vi "CheckStoped.vi"(0 "OSC in":refnum<visa-resource-name>, 1 "error in (no error)":errorcluster) -> (2 "OSC out":refnum<visa-resource-name>, 3 "Stopped?":bool, 4 "error out":errorcluster)   [LabVIEW 2016]
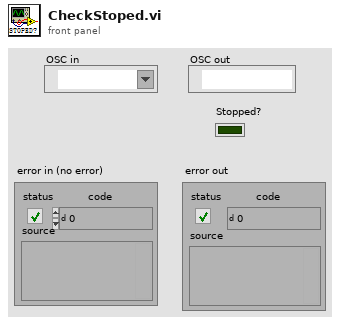
[diagram p1: front panel]
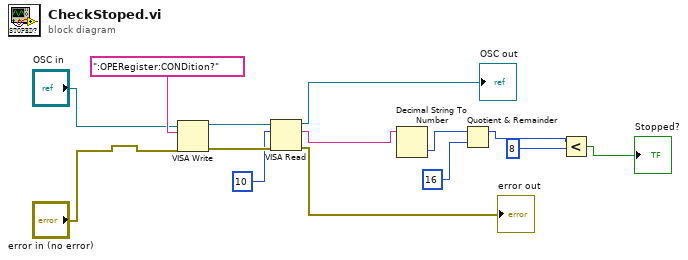
[diagram p0: block diagram]
diagram:
  n1 = VISA Write(VISA resource name="OSC in", write buffer=":OPERegister:CONDition?", error in (no error)="error in (no error)") -> (VISA resource name out=w13:refnum<visa-resource-name>, error out=w12:errorcluster)  [unwired: 1 out]
  n2 = VISA Read(VISA resource name=w13, byte count=10, error in (no error)=w12) -> (VISA resource name out=→"OSC out":refnum<visa-resource-name>, read buffer=w8:string, error out=→"error out":errorcluster)  [unwired: 1 out]
  n3 = Decimal String To Number(string=w8) -> (number=w7:i32)  [unwired: 2 in, 1 out]
  n4 = Quotient & Remainder(x=w7, y=16) -> (x-y*floor(x/y)=w5:i32)  [unwired: 1 out]
  n5 = Less?(x=w5, y=8) -> (x < y?=→"Stopped?":bool)
